vi "Enable PPSU 2.vi"() -> (0 "error Out":errorcluster, 1 "Device information":string[](array[string]), 2 "Device information array":string[][](array[string]), 3 "PPSU IP String":string)   [LabVIEW 2022 SP3]
uses:
  Controls/ALL Health.ctl
  6D_Global.vi
panel:
  out "Data of the initialized master":string[](array[string])
  out ".not. x?":bool
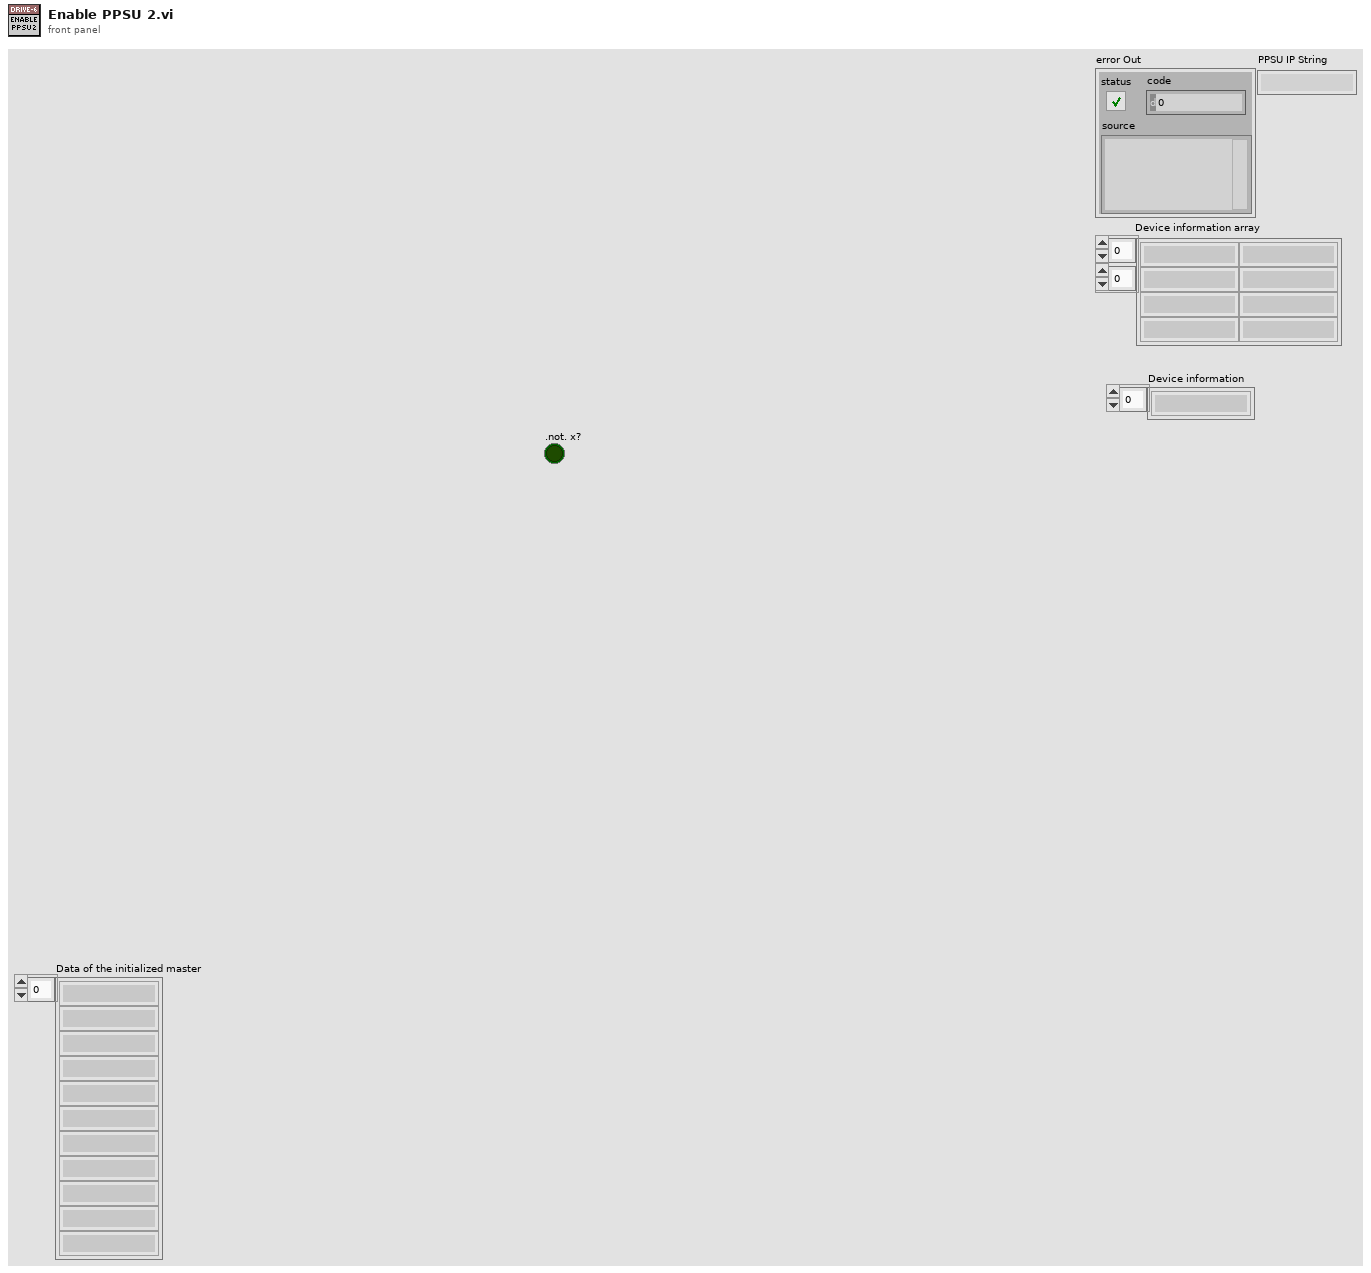
[diagram p1: front panel]
types:
  T1 = cluster{"Start IP":u8[], "Stop IP":u8[], "port":u16}
  T2 = typedef "ALL Health.ctl" = enum16{"DO HS", "Datalog HS", "PPSU HS", "PPSU 2 HS ", "ETH_1", "ETH_2", "ETH_3", "ETH_4", "ETH_5", "ETH_6", "ETH_7", "ETH_8", "ETH_9", "ETH_10", "ETH_11", "ETH_12"}
  T3 = enum16{"Init", "Read 'All'", "Read 'n'", "Read '1'", "Write '1'", "Write 'n'", "Write 'All'"}
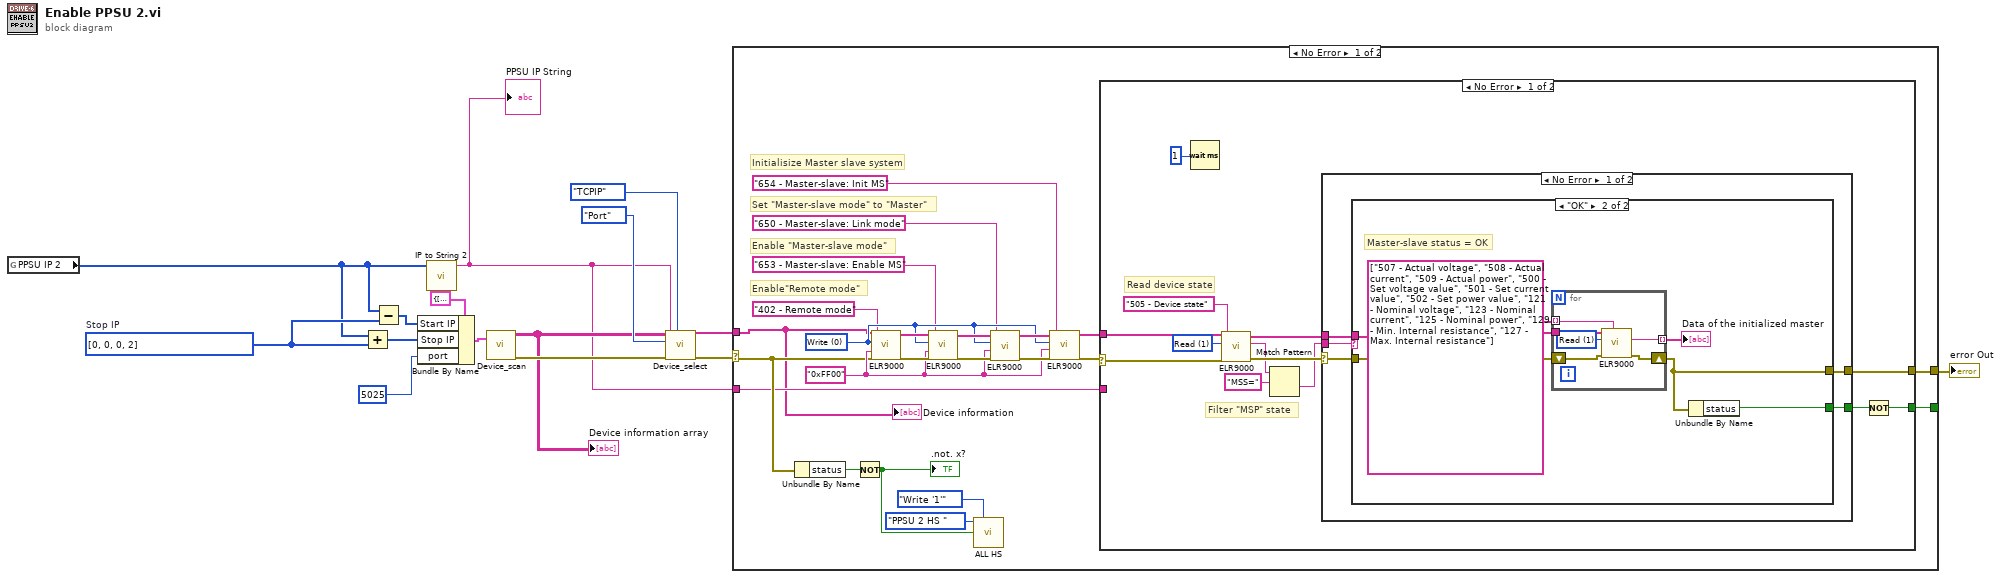
[diagram p0: block diagram]
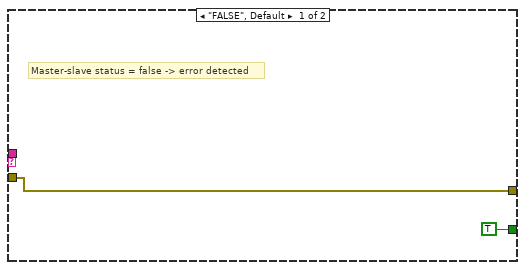
[diagram p2: hidden frame]
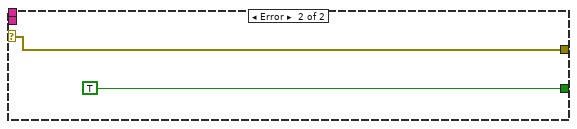
[diagram p3: hidden frame]
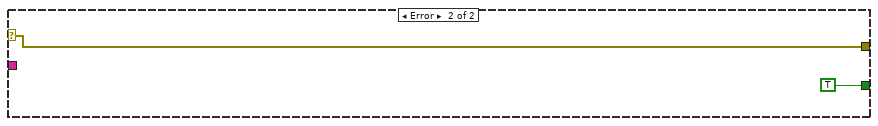
[diagram p4: hidden frame]
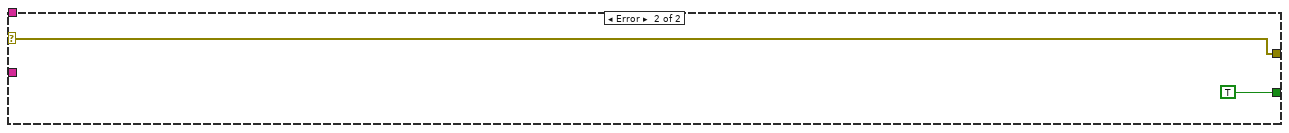
[diagram p5: hidden frame]
diagram:
  w4 = u8[] [0, 0, 0, 2]  # Stop IP
  n1 = global read "6D_Global.vi" "PPSU IP 2"() -> (w1:u8[])
  n2 = Add(x=w1, y=w4) -> (x+y=w6:u8[])
  n3 = Subtract(x=w1, y=w4) -> (x-y=w5:u8[])
  n4 = Bundle By Name(cluster=T1 {"Start IP"=[], "Stop IP"=[], "port"=0}, "Start IP"=w5, "Stop IP"=w6, "port"=u16 5025) -> (w9:T1)
  n5 = call "IP to String 2.vi"("Start IP"=w1) -> ("resulting string"=w2:string)  [unwired: 10 in]
  "PPSU IP String" <- w2
  n6 = call <instrlib>:"Device_scan.vi"("IP settings"=w9) -> ("Device information array"=w3:string[][], "error out"=w8:errorcluster)  [unwired: 1 in, 2 out]
  "Device information array" <- w3
  n7 = call <instrlib>:"Device_select.vi"("Reference"=enum16{"ASRL/COM", "GPIB", "TCPIP"}."TCPIP", "error in (no error)"=w8, "Alias"=w2, "Open by"=enum16{"Device Node", "Serial number", "Port"}."Port", "Device information array"=w3) -> ("error out"=w14:errorcluster, "Device information"=w15:string[])  [unwired: 2 in]
  n8 = case shown="No Error" w14 {
    selector: w14 -> [w23 w75]
    tunnel: [w34 TRUE] -> _
    tunnel: w15 -> [w16 _]
    tunnel: w2 -> [w21 _]
    tunnel: [w20 w75] -> w12
    frame No Error {
      w28 = u8 0 items=["Write", "Read"] ("Access")
      w29 = "0xFF00" ("Value")
      # "Initialisize Master slave system"
      # "Set \"Master-slave mode\" to \"Master\""
      # "Enable \"Master-slave mode\""
      # "Enable\"Remote mode\""
      n9 = Unbundle By Name(w23) -> ("status"=w22:bool)
      n10 = Not(x=w22) -> (.not. x?=w17:bool)
      ".not. x?" <- w17
      n11 = call <instrlib>:"ELR9000.vi"("Command list"="402 - Remote mode", "Error in"=w23, "Value"=w29, "Access"=w28, "Device information in"=w16) -> ("Error out"=w36:errorcluster, "Device information out"=w35:string[])  [unwired: 1 in, 2 out]
      n12 = call <instrlib>:"ELR9000.vi"("Command list"="653 - Master-slave: Enable MS", "Error in"=w36, "Value"=w29, "Access"=w28, "Device information in"=w35) -> ("Error out"=w33:errorcluster, "Device information out"=w30:string[])  [unwired: 1 in, 2 out]
      n13 = call "ALL HS.vi"("Loop"=ALL_Health."PPSU 2 HS ", "Option"=T3."Write '1'", "Status"=w17) -> ()  [unwired: 10 in, 3 out]
      n14 = call <instrlib>:"ELR9000.vi"("Command list"="650 - Master-slave: Link mode", "Error in"=w33, "Value"=w29, "Access"=w28, "Device information in"=w30) -> ("Error out"=w32:errorcluster, "Device information out"=w31:string[])  [unwired: 1 in, 2 out]
      n15 = call <instrlib>:"ELR9000.vi"("Command list"="654 - Master-slave: Init MS", "Error in"=w32, "Value"=w29, "Access"=w28, "Device information in"=w31) -> ("Error out"=w38:errorcluster, "Device information out"=w37:string[])  [unwired: 1 in, 2 out]
      n16 = case shown="No Error" w38 {
        selector: w38 -> [w41 w73]
        tunnel: w37 -> [w40 _]
        tunnel: [w51 TRUE] -> w34
        tunnel: w21 -> [_ _]
        tunnel: [w39 w73] -> w20
        frame No Error {
          w50 = u8 1 items=["Write", "Read"] ("Access")
          # "Read device state"
          # "Filter \"MSP\" state"
          n17 = Wait (ms)(milliseconds to wait=u32 1 ("Zu wartende ms")) -> ()  [unwired: 1 out]
          n18 = call <instrlib>:"ELR9000.vi"("Command list"="505 - Device state", "Error in"=w41, "Access"=w50, "Device information in"=w40) -> ("Error out"=w49:errorcluster, "Read data"=w47:string, "Device information out"=w48:string[])  [unwired: 2 in, 1 out]
          n19 = Match Pattern(string=w47, regular expression="MSS=" ("regulärer Ausdruck")) -> (after substring=w44:string)  [unwired: 1 in, 3 out]
          n20 = case shown="No Error" w49 {
            selector: w49 -> [w54 w71]
            tunnel: w44 -> [w56 _]
            tunnel: w48 -> [w55 _]
            tunnel: [w53 TRUE] -> w45
            tunnel: [w52 w71] -> w39
            frame No Error {
              n21 = case shown="\"OK\"" w56 {
                tunnel: w55 -> [_ w63]
                tunnel: w54 -> [w57 w62]
                tunnel: [TRUE w61] -> w53
                tunnel: [w57 w59] -> w52
                frame "FALSE", Default {
                  # "Master-slave status = false -> error detected"
                }
                frame "OK" {
                  # "Master-slave status = OK"
                  n22 = for {
                    tunnel: w63 -> [w70]
                    tunnel: string[] ["507 - Actual voltage", "508 - Actual current", "509 - Actual power", "500 - Set voltage value", "501 - Set current value", "502 - Set power value", "121 - Nominal voltage", "123 - Nominal current", "125 - Nominal power", "129 - Min. Internal resistance", "127 - Max. Internal resistance"] -> [w68] mode=indexing
                    shift-right: [w66] -> w59
                    shift-left: w62 -> [w67]
                    tunnel: [w65] -> w64 mode=indexing
                    w69 = u8 1 items=["Write", "Read"] ("Access")
                    n23 = call <instrlib>:"ELR9000.vi"("Command list"=w68, "Error in"=w67, "Access"=w69, "Device information in"=w70) -> ("Error out"=w66:errorcluster, "Read data"=w65:string)  [unwired: 2 in, 2 out]
                  }
                  "Data of the initialized master" <- w64
                  n24 = Unbundle By Name(w59) -> ("status"=w61:bool)
                }
              }
            }
            frame Error {
            }
          }
          n25 = Not(x=w45) -> (.not. x?=w51:bool)
        }
        frame Error {
        }
      }
      "Device information" <- w16
    }
    frame Error {
    }
  }
  "error Out" <- w12
